vi "Template Tool.vi"() -> ()   [LabVIEW 2019]
doc: "This tool oplens a copy from Template.vilib"
uses:
  <vilib>/LabVIEW Icon API/API_Rectangle Colors.ctl
  <vilib>/LabVIEW Icon API/lv_icon/Classes/Icon/Icon.lvclass
  <vilib>/LabVIEW Icon API/API_Rectangle Dimension.ctl
  <vilib>/LabVIEW Icon API/API_Text.ctl
  <vilib>/LabVIEW Icon API/API_Test Settings.ctl
  <vilib>/LabVIEW Icon API/lv_icon/Controls/Alignment.ctl
  <vilib>/LabVIEW Icon API/API_Text Colors.ctl
  <vilib>/LabVIEW Icon API/LabVIEW Icon API.lvlib
panel:
  out "error out":errorcluster
  in  "Error In":errorcluster
  out "VI Icon Template":picture
  out "Template found":bool
  in  "Icon BG Color":u32(colorbox)=9567230
  in  "Module Name":string="Test"
  # "#TODO: Change this simple VI to an Assistant."
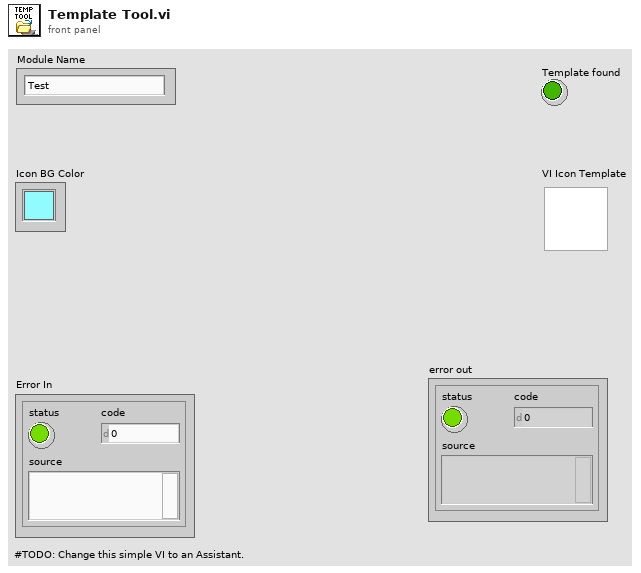
[diagram p1: front panel]
types:
  T1 = typedef "LabVIEW Icon API.lvlib/API_Test Settings.ctl" = cluster{"Font":string, "Alignment":T2, "Size":u8, "Center text":bool, "Capitalize text":bool, "Text color":T3}
  T2 = typedef "Alignment.ctl" = u16
  T3 = typedef "LabVIEW Icon API.lvlib/API_Text Colors.ctl" = cluster{"Line 1 color":u32, "Line 2 color":u32, "Line 3 color":u32, "Line 4 color":u32}
  T4 = typedef "LabVIEW Icon API.lvlib/API_Text.ctl" = cluster{"Line 1 text":string, "Line 2 text":string, "Line 3 text":string, "Line 4 text":string}
  T5 = typedef "LabVIEW Icon API.lvlib/API_Rectangle Dimension.ctl" = cluster{"Width":i16, "Height":i16}
  T6 = typedef "LabVIEW Icon API.lvlib/API_Rectangle Colors.ctl" = cluster{"Border":u32, "Background":u32}
  T7 = typedef "imagedata.ctl" = cluster{"image type":i32, "image depth":i32, "image":u8[], "mask":u8[], "colors":u32[], "Rectangle":cluster{"left":i16, "top":i16, "right":i16, "bottom":i16}}
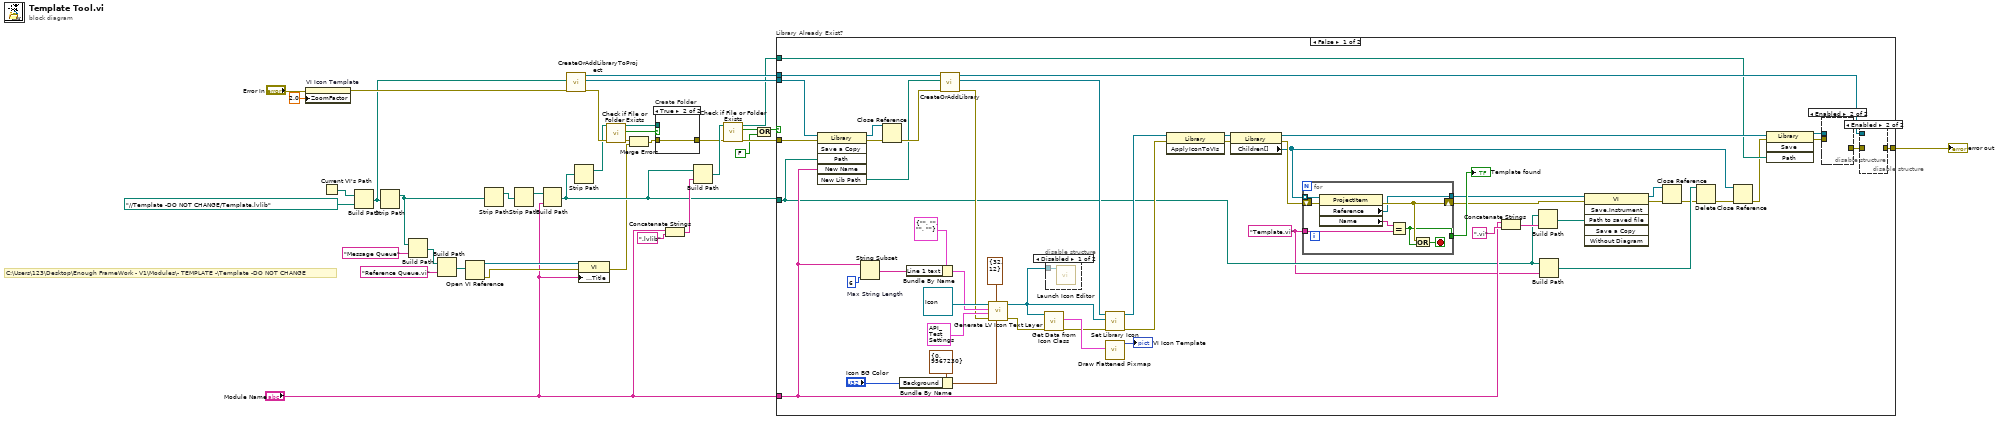
[diagram p0: block diagram]
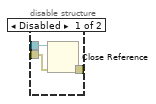
[diagram p2: hidden frame]
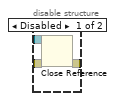
[diagram p3: hidden frame]
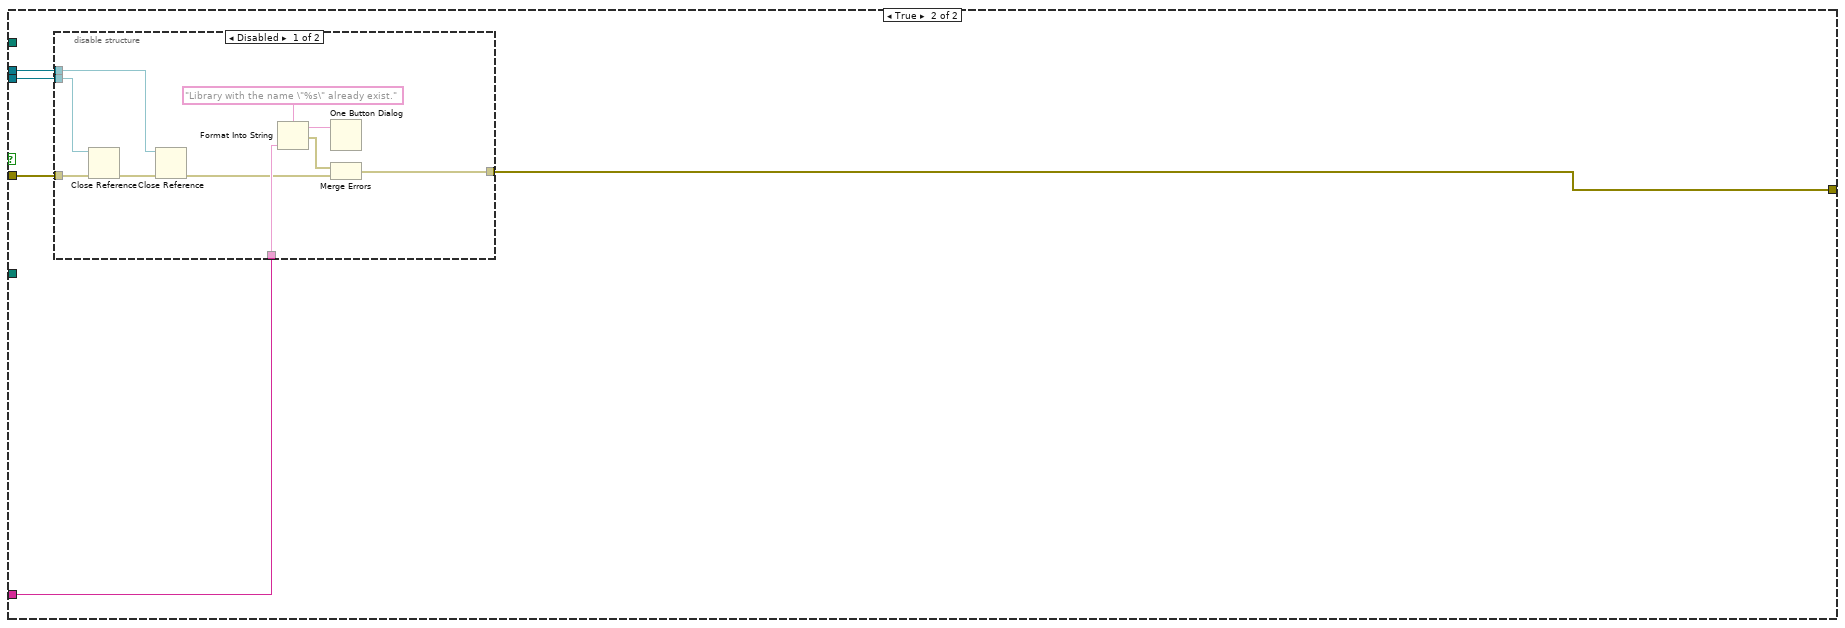
[diagram p5: hidden frame]
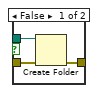
[diagram p7: hidden frame]
diagram:
  # "C:\\Users\\123\\Desktop\\Enough FrameWork - V1\\Modules\\- TEMPLATE -\\Template -DO NOT CHANGE"
  n1 = property on="VI Icon Template" class="Pict"(error in="Error In", "ZoomFactor"=sgl 2.0 ("Zoom Factor")) -> (error out=w20:errorcluster)  [unwired: 1 in, 1 out]
  n2 = Current VI's Path() -> (path=w15:path)
  n3 = Build Path(base path=w15, name or relative path=path "../../Template -DO NOT CHANGE/Template.lvlib" ("stripped path")) -> (appended path=w16:path)
  n4 = Strip Path(path=w16) -> (stripped path=w11:path)  [unwired: 1 out]
  n5 = Build Path(base path=w11, name or relative path="Message Queue") -> (appended path=w9:path)
  n6 = Build Path(base path=w9, name or relative path="Reference Queue.vi") -> (appended path=w7:path)
  n7 = Open VI Reference(vi path=w7) -> (vi reference=w6:refnum<vi>, error out=w5:errorcluster)  [unwired: 5 in]
  n8 = Strip Path(path=w11) -> (stripped path=w27:path)  [unwired: 1 out]
  n9 = Strip Path(path=w27) -> (stripped path=w18:path)  [unwired: 1 out]
  n10 = Build Path(base path=w18, name or relative path="Module Name") -> (appended path=w25:path)
  n11 = call <vilib>:"CreateOrAddLibraryToProject.vi"("error in (no error)"=w20, "Library Path In (Create New)"=w16) -> ("error out"=w32:errorcluster, "Library Reference Out"=w33:refnum<vi>, "Project Reference Out"=w31:refnum<vi>)  [unwired: 1 in, 6 out]
  n12 = Strip Path(path=w25) -> (stripped path=w23:path)  [unwired: 1 out]
  n13 = property class="VI"(reference=w6, error in=w5, "Front Panel.Title"="Module Name") -> (error out=w2:errorcluster)  [unwired: 1 out]
  n14 = call <vilib>:"Check if File or Folder Exists.vi"("error in (no error)"=w32, "path"=w23) -> ("error out"=w35:errorcluster, "file or folder exists?"=w36:bool, "dup path"=w34:path)  [unwired: 7 out]
  n15 = Merge Errors(w35, w2) -> (w3:errorcluster)
  n16 = case "Create Folder" shown="True" w36 {
    tunnel: w3 -> [w39 w40]
    tunnel: [w38 w40] -> w26
    tunnel: w34 -> [w37 _]
    frame False {
      n17 = Create Folder(path (use dialog)=w37, error in=w39) -> (error out=w38:errorcluster)  [unwired: 3 out]
    }
    frame True {
    }
  }
  n18 = Concatenate Strings("Module Name", ".lvlib" ("string")) -> (w29:string)
  n19 = Build Path(base path=w25, name or relative path=w29) -> (appended path=w30:path)
  n20 = call <vilib>:"Check if File or Folder Exists.vi"("error in (no error)"=w26, "path"=w30) -> ("error out"=w24:errorcluster, "file or folder exists?"=w14:bool, "dup path"=w22:path)  [unwired: 7 in]
  n21 = Or(x=w14, y=FALSE) -> (x .or. y?=w13:bool)
  n22 = case "Library Already Exist?" shown="False" w13 {
    tunnel: w33 -> [w92 w110]
    tunnel: w31 -> [w74 w109]
    tunnel: w25 -> [w43 _]
    tunnel: "Module Name" -> [w44 w112]
    tunnel: w24 -> [w69 w108]
    tunnel: [w66 w111] -> w1
    tunnel: w22 -> [w57 _]
    frame False {
      w41 = "Template.vi" ("VI Name")
      w79 = 6  # Max String Length
      n23 = invoke class="Library" method="Save a Copy"(reference=w92, error in=w69, "Path"=w43, "New Name"=w44) -> (reference out=w72:refnum<vi>, error out=w75:errorcluster, "New Lib Path"=w65:path)  [unwired: 2 in, 3 out]
      n24 = String Subset(string=w44, length (rest)=w79) -> (substring=w80:string)  [unwired: 1 in]
      n25 = Close Reference(reference=w72, error in (no error)=w75) -> (error out=w68:errorcluster)
      n26 = Bundle By Name(cluster=T6 {"Border"=0, "Background"=9567230} ("Rectangle colors (black, white)"), "Background"="Icon BG Color") -> (w90:T6)
      n27 = Bundle By Name(cluster=T4 {"Line 1 text"="", "Line 2 text"="", "Line 3 text"="", "Line 4 text"=""} ("Text"), "Line 1 text"=w80) -> (w81:T4)
      n28 = call-poly <vilib>:"CreateOrAddLibrary.vi"("error in (no error)"=w68, "Library Path In (Create New)"=w65, "Project Reference In (Create New)"=w74) -> ("error out"=w67:errorcluster, "Library Reference Out"=w71:refnum<vi>, "Project Reference Out"=w73:refnum<vi>)  [unwired: 6 in]
      n29 = call <vilib>:"Generate LV Icon Text Layer.vi"("Rectangle colors (black, white)"=w90, "Rectangle dimension (32,32)"=T5 {"Width"=32, "Height"=12}, "error in (no error)"=w67, "Text settings"=T1 {"Font"="Small Fonts", "Alignment"=1, "Size"=8, "Center text"=TRUE, "Capitalize text"=TRUE, "Text color"={"Line 1 color"=0, "Line 2 color"=0, "Line 3 color"=0, "Line 4 color"=0}}, "Text"=w81, "Icon in"=refnum<class "Icon.lvclass"> refnum ("Icon.lvclass in")) -> ("error out"=w55:errorcluster, "Icon out"=w53:refnum<class "Icon.lvclass">)  [unwired: 4 in]
      n30 = call <vilib>:"Get Data from Icon Class.vi"("error in (no error)"=w55, "Icon in"=w53) -> ("error out"=w54:errorcluster, "Color Image Data"=w56:T7)  [unwired: 6 in, 2 out]
      n31 = disable-structure shown="Disabled" {
        disable-tunnel: w53 -> [w99 _]
        frame Disabled {
          n32 = call <vilib>:"Launch Icon Editor.vi"("Icon in"=w99) -> ()  [unwired: 8 in, 3 out]
        }
        frame Enabled {
        }
      }
      n33 = call <vilib>:"Set Library Icon.vi"("error in (no error)"=w54, "Icon"=w53, "Library Refnum in"=w71) -> ("error out"=w84:errorcluster, "Library Refnum out"=w85:refnum<vi>)  [unwired: 7 in]
      n34 = call <vilib>:"Draw Flattened Pixmap.vi"("image data"=w56) -> ("new picture"=→"VI Icon Template":picture)  [unwired: 8 in]
      n35 = invoke class="Library" method="ApplyIconToVIs"(reference=w85, error in=w84) -> (reference out=w46:refnum<vi>, error out=w58:errorcluster)  [unwired: 1 in, 1 out]
      n36 = property class="Library"(reference=w46, error in=w58) -> (reference out=w63:refnum<vi>, error out=w70:errorcluster, "Children[]"=w45:refnum<vi>[])
      n37 = for {
        tunnel: w45 -> [w107] mode=indexing
        tunnel: [w101] -> w62
        tunnel: w41 -> [w106]
        tunnel: [w102] -> w77
        shift-right: [w103] -> w64
        shift-left: w70 -> [w104]
        stop <- w105 stop-if-true
        n38 = property class="ProjectItem"(reference=w107, error in=w104) -> (error out=w103:errorcluster, "Reference"=w101:refnum<vi>, "Name"=w100:string)  [unwired: 1 out]
        n39 = Equal?(x=w100, y=w106) -> (x = y?=w102:bool)
        n40 = Or(x=w103, y=w102) -> (x .or. y?=w105:bool)
      }
      "Template found" <- w77
      n41 = Concatenate Strings(w44, ".vi" ("string")) -> (w61:string)
      n42 = Build Path(base path=w43, name or relative path=w61) -> (appended path=w50:path)
      n43 = Build Path(base path=w43, name or relative path=w41) -> (appended path=w76:path)
      n44 = invoke class="VI" method="Save.Instrument"(reference=w62, error in=w64, "Path to saved file"=w50) -> (reference out=w51:refnum<vi>, error out=w49:errorcluster)  [unwired: 3 in, 4 out]
      n45 = Close Reference(reference=w51, error in (no error)=w49) -> (error out=w48:errorcluster)
      n46 = Delete(path (use dialog)=w76, error in=w48) -> (error out=w42:errorcluster)  [unwired: 3 in, 2 out]
      n47 = Close Reference(reference=w45, error in (no error)=w42) -> (error out=w47:errorcluster)
      n48 = invoke class="Library" method="Save"(reference=w63, error in=w47, "Path"=w57) -> (reference out=w60:refnum<vi>, error out=w59:errorcluster)  [unwired: 1 in, 2 out]
      n49 = disable-structure shown="Enabled" {
        disable-tunnel: [w95 _] -> w88
        disable-tunnel: w60 -> [w94 _]
        disable-tunnel: w59 -> [w93 _]
        frame Disabled {
          n50 = Close Reference(reference=w94, error in (no error)=w93) -> (error out=w95:errorcluster)
        }
        frame Enabled {
        }
      }
      n51 = disable-structure shown="Enabled" {
        disable-tunnel: w88 -> [w98 _]
        disable-tunnel: w73 -> [w97 _]
        disable-tunnel: [w96 _] -> w66
        frame Disabled {
          n52 = Close Reference(reference=w97, error in (no error)=w98) -> (error out=w96:errorcluster)
        }
        frame Enabled {
        }
      }
    }
    frame True {
      n53 = disable-structure shown="Disabled" {
        disable-tunnel: w112 -> [w122 _]
        disable-tunnel: [w121 _] -> w111
        disable-tunnel: w110 -> [w117 _]
        disable-tunnel: w109 -> [w116 _]
        disable-tunnel: w108 -> [w115 _]
        frame Disabled {
          n54 = Close Reference(reference=w117, error in (no error)=w115) -> (error out=w114:errorcluster)
          n55 = Close Reference(reference=w116, error in (no error)=w114) -> (error out=w113:errorcluster)
          n56 = Format Into String(format string="Library with the name \"%s\" already exist." ("initial string"), w122) -> (resulting string=w119:string, error out=w120:errorcluster)  [unwired: 2 in]
          n57 = One Button Dialog(message=w119) -> ()  [unwired: 1 in, 1 out]
          n58 = Merge Errors(w120, w113) -> (w121:errorcluster)
        }
        frame Enabled {
        }
      }
    }
  }
  "error out" <- w1
